vi "test_simple_Doppler.vi"() -> ()   [LabVIEW 2009]
doc: "Copyright (C) 2009, Stepan A. Baranov\nweb: http://www.OCTLab.org/\nemail: stepan@baranov.su"
uses:
  OCTLib.dll
panel:
  out "error out":errorcluster
  out "width":i32
  out "height":i32
  in  "Small/Big":bool
  out "loop #":i32
  out "RSM_STAT time":u32
  out "LabView time":u32
  out "RSM_STAT Array":dbl[][](array[numeric])
  out "LabView Array":dbl[][](array[numeric])
  in  "stop":bool
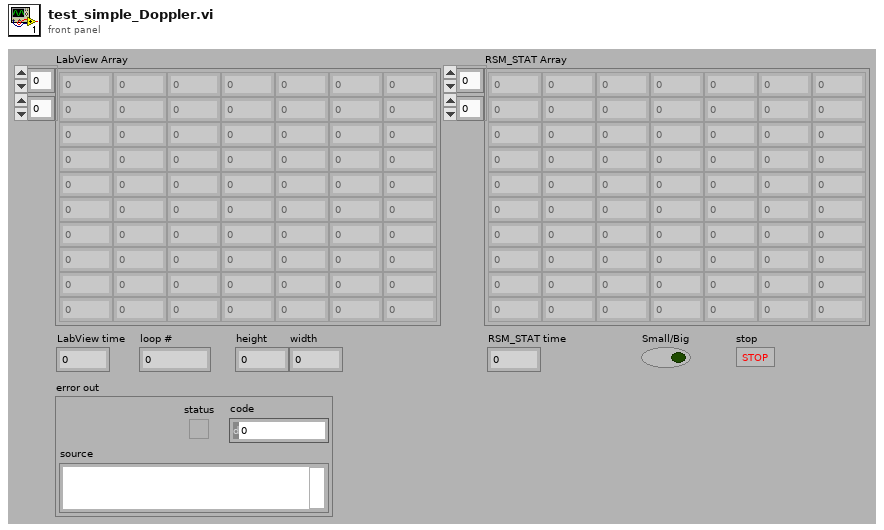
[diagram p1: front panel]
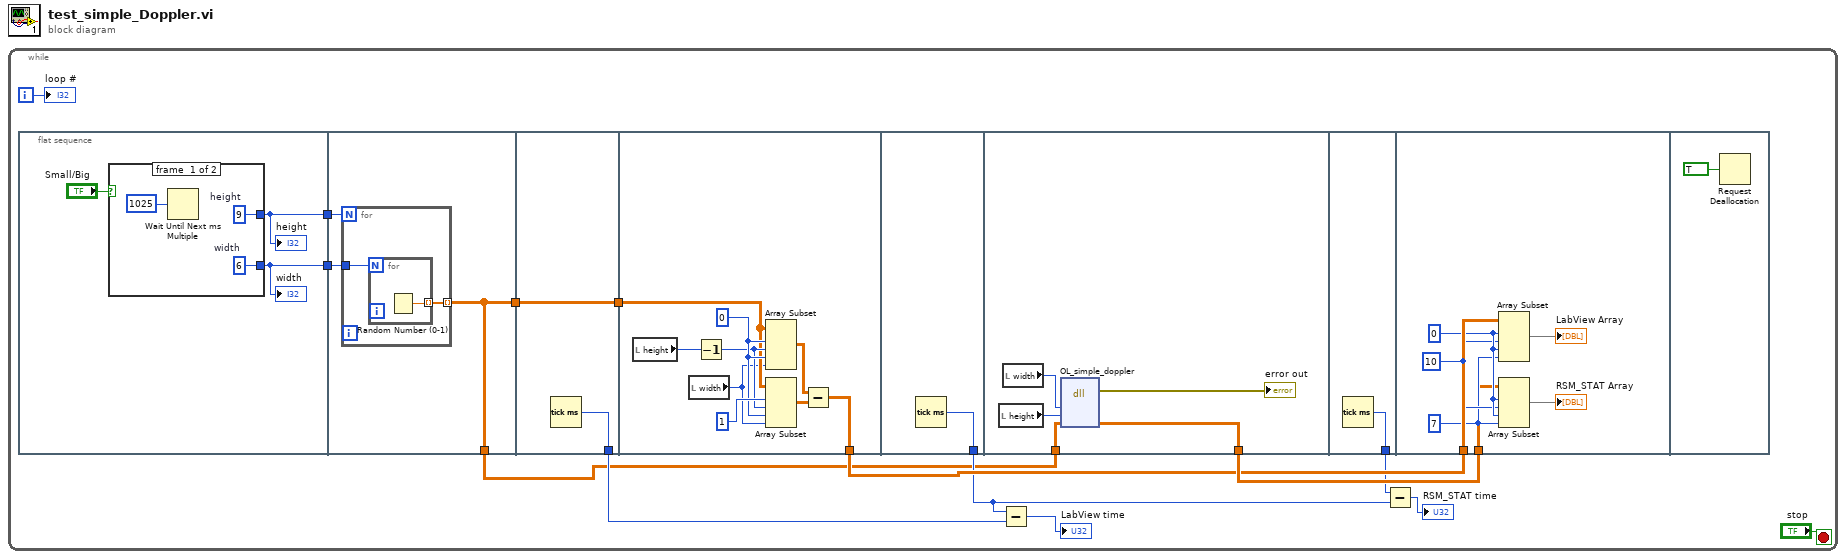
[diagram p0: block diagram]
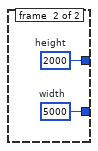
[diagram p2: hidden frame]
diagram:
  n1 = while {
    i -> [w6]
    stop <- "stop" stop-if-true
    n2 = flat-sequence {
      tunnel: [w16] -> w2
      tunnel: [w15] -> w1
      tunnel: [w23] -> w5
      tunnel: [w23] -> w3
      tunnel: w2 -> [w25]
      tunnel: w1 -> [w24]
      tunnel: [w30] -> w11
      tunnel: [w29] -> w4
      tunnel: w3 -> [w29]
      tunnel: [w33] -> w12
      tunnel: w4 -> [w34]
      tunnel: [w40] -> w8
      tunnel: w5 -> [w43]
      tunnel: [w42] -> w13
      tunnel: [w46] -> w9
      tunnel: w13 -> [w47]
      tunnel: w12 -> [w53]
      frame #0 {
        n3 = case shown="True" "Small/Big" {
          tunnel: [w19 w22] -> w15
          tunnel: [w20 w21] -> w16
          frame #0 {
            w20 = 6  # width
            w19 = 9  # height
            n4 = Wait Until Next ms Multiple(millisecond multiple=u32 1025) -> ()  [unwired: 1 out]
          }
          frame #1 {
            w21 = 5000  # width
            w22 = 2000  # height
          }
        }
        "height" <- w15
        "width" <- w16
      }
      frame #1 {
        n5 = for {
          N: w24 -> [_]
          tunnel: w25 -> [w27]
          tunnel: [w26] -> w23 mode=indexing
          n6 = for {
            N: w27 -> [_]
            tunnel: [w28] -> w26 mode=indexing
            n7 = Random Number (0-1)() -> (number: 0 to 1=w28:dbl)
          }
        }
      }
      frame #2 {
        n8 = Tick Count (ms)() -> (millisecond timer value=w30:u32)
      }
      frame #3 {
        w38 = 0 ("index")
        n9 = local read "height"() -> (w32:i32)
        n10 = local read "width"() -> (w31:i32)
        n11 = Decrement(x=w32) -> (x-1=w37:i32)
        n12 = Array Subset(array=w34, index (row)=w38, length (row)=w37, index (col)=w38, length (col)=w31) -> (w36:dbl[][])
        n13 = Array Subset(array=w34, index (row)=1 ("index"), length (row)=w37, index (col)=w38, length (col)=w31) -> (w35:dbl[][])
        n14 = Subtract(x=w36, y=w35) -> (x-y=w33:dbl[][])
      }
      frame #4 {
        n15 = Tick Count (ms)() -> (millisecond timer value=w40:u32)
      }
      frame #5 {
        n16 = local read "height"() -> (w44:i32)
        n17 = local read "width"() -> (w45:i32)
        n18 = dll-call lib="OCTLib.dll" fn="OL_simple_doppler"("width"=w45, "height"=w44, "data"=w43) -> (error out=→"error out":errorcluster, "data"=w42:dbl[][])  [unwired: 6 in, 1 out]
      }
      frame #6 {
        n19 = Tick Count (ms)() -> (millisecond timer value=w46:u32)
      }
      frame #7 {
        w50 = 10 ("length")
        w49 = 7 ("length")
        w51 = 0 ("index")
        n20 = Array Subset(array=w53, index (row)=w51, length (row)=w50, index (col)=w51, length (col)=w49) -> (→"LabView Array":dbl[][])
        n21 = Array Subset(array=w47, index (row)=w51, length (row)=w50, index (col)=w51, length (col)=w49) -> (→"RSM_STAT Array":dbl[][])
      }
      frame #8 {
        n22 = Request Deallocation(TRUE ("flag")) -> ()
      }
    }
    n23 = Subtract(x=w8, y=w11) -> (x-y=→"LabView time":u32)
    n24 = Subtract(x=w9, y=w8) -> (x-y=→"RSM_STAT time":u32)
    "loop #" <- w6
  }
